vi "Test Line Filter.vi"(8 "error in (no error)":errorcluster, 11 "VISA resource name":refnum<visa-resource-name>) -> (0 "error out":errorcluster, 3 "VISA resource name":refnum<visa-resource-name>)   [LabVIEW 2019, in "SR7270 Drivers.lvlib"]
uses:
  SR7270 Drivers.lvlib
  Typedefs/LF--enum.ctl
  <vilib>/addons/_JKI Toolkits/Caraya/classes/Assert/Assert.lvclass
  <vilib>/addons/_JKI Toolkits/Caraya/classes/Test/Test.lvclass
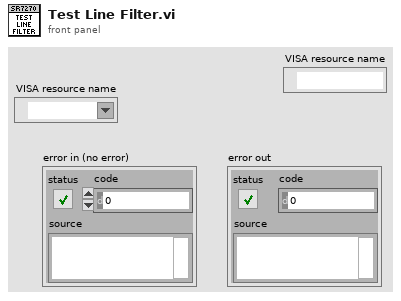
[diagram p1: front panel]
types:
  T1 = typedef "SR7270 Drivers.lvlib/LF--enum.ctl" = enum16{"Off", "60 Hz", "120 Hz", "60 & 120 Hz"}
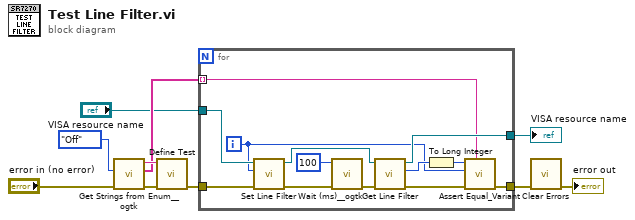
[diagram p0: block diagram]
diagram:
  n1 = call <userlib>:"Get Strings from Enum__ogtk.vi"("error in (no error)"="error in (no error)", "Enum"=LF--enum."Off" ("Line Frequency Rejection")) -> ("error out"=w5:errorcluster, "Enum Strings"=w3:string[], "Enum Name"=w4:string)  [unwired: 6 in, 1 out]
  n2 = call <vilib>:"Define Test.vi"("error in (no error)"=w5, "Label (VI Title)"=w4) -> ("error out"=w10:errorcluster)  [unwired: 9 in]
  n3 = for {
    tunnel: "VISA resource name" -> [w22]
    tunnel: w10 -> [w14]
    tunnel: [w20] -> w9
    tunnel: [w19] -> w1
    tunnel: w3 -> [w11] mode=indexing
    i -> [w12]
    n4 = call "Set Line Filter.vi"("error in (no error)"=w14, "Line Frequency Rejection"=w12, "VISA resource name"=w22) -> ("error out"=w16:errorcluster, "VISA resource name out"=w23:refnum<visa-resource-name>)  [unwired: 7 in]
    n5 = call <userlib>:"Wait (ms)__ogtk.vi"("error in (no error)"=w16, "milliseconds to wait"=u32 100) -> ("error out"=w18:errorcluster)  [unwired: 8 in, 1 out]
    n6 = call "Get Line Filter.vi"("error in (no error)"=w18, "VISA resource name"=w23) -> ("error out"=w21:errorcluster, "Line Frequency Rejection"=w15:T1, "VISA resource name out"=w19:refnum<visa-resource-name>)  [unwired: 7 in]
    n7 = To Long Integer(number=w15) -> (32bit integer=w13:i32)
    n8 = call <vilib>:"Assert Equal_Variant.vi"("Label"=w11, "error in (no error)"=w21, "Y"=w12, "X"=w13) -> ("error out"=w20:errorcluster)  [unwired: 7 in]
  }
  "VISA resource name" <- w1
  n9 = call <vilib>:"Clear Errors.vi"("error in (no error)"=w9) -> ("error out"=→"error out":errorcluster)  [unwired: 5 in, 1 out]
